vi "CRYASIO Play Buffer.vi"(6 "Gen Idx":u32, 7 "is Main":bool, 8 "Limit":u32, 9 "Buffer Amount":u32, 10 "Buffer Index":u32, 11 "Data Array":sgl[](array[numeric])) -> (0 "Buffer Amount Out":u32, 1 "Buffer Index Out":u32)   [LabVIEW 2013]
uses:
  CRYMisc vis settings global.vi
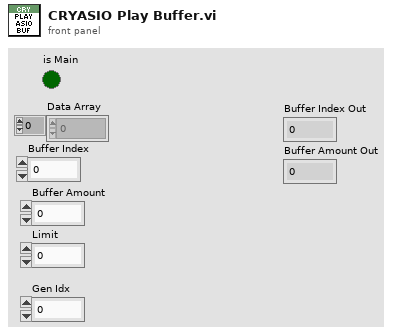
[diagram p1: front panel]
types:
  T1 = cluster{"Gen Idx":i32, "Chn Idx":i32, "Data":sgl[]}[]
  T2 = cluster{"Gen Idx":i32, "Chn Idx":i32, "Data":sgl[]}
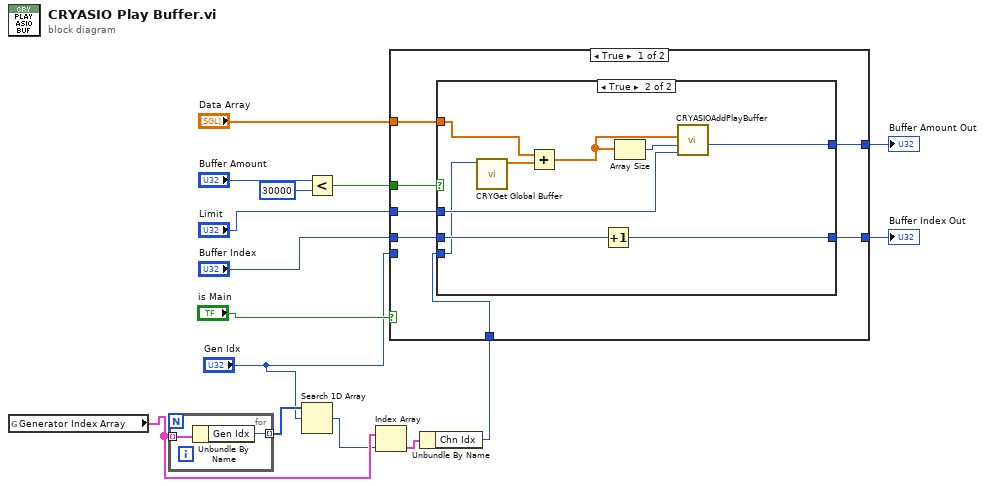
[diagram p0: block diagram]
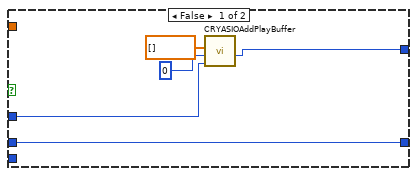
[diagram p2: hidden frame]
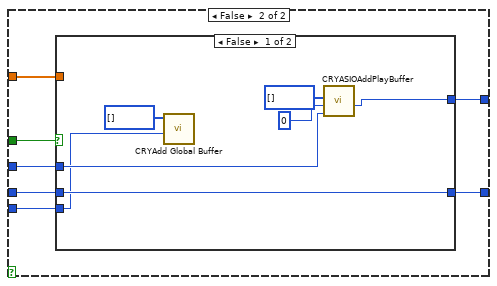
[diagram p3: hidden frame]
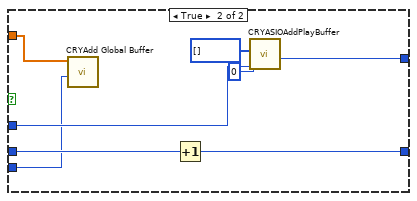
[diagram p4: hidden frame]
diagram:
  n1 = global read "CRYMisc vis settings global.vi" "Generator Index Array"() -> (w4:T1)
  n2 = for {
    tunnel: w4 -> [w17] mode=indexing
    tunnel: [w16] -> w6 mode=indexing
    n3 = Unbundle By Name(w17) -> ("Gen Idx"=w16:i32)
  }
  n4 = Search 1D Array(1D array=w6, element="Gen Idx") -> (index of element=w3:i32)  [unwired: 1 in]
  n5 = Less?(x="Buffer Amount", y=u32 30000) -> (x < y?=w13:bool)
  n6 = Index Array(array=w4, index=w3) -> (element=w2:T2)
  n7 = Unbundle By Name(w2) -> ("Chn Idx"=w1:i32)
  n8 = case shown="True" "is Main" {
    tunnel: w13 -> [w24 w45]
    tunnel: "Data Array" -> [w23 w44]
    tunnel: "Buffer Index" -> [w22 w43]
    tunnel: [w21 w42] -> w10
    tunnel: "Limit" -> [w20 w41]
    tunnel: [w19 w40] -> w8
    tunnel: "Gen Idx" -> [_ w39]
    tunnel: w1 -> [w18 _]
    frame True {
      n9 = case shown="True" w24 {
        tunnel: w23 -> [_ w31]
        tunnel: w22 -> [w29 w38]
        tunnel: [w29 w37] -> w21
        tunnel: w20 -> [w26 w35]
        tunnel: [w25 w34] -> w19
        tunnel: w18 -> [_ w33]
        frame False {
          n10 = call "CRYASIOAddPlayBuffer.vi"("Limit"=w26, "Data Length"=0, "pData"=sgl[] []) -> ("Buffer Amount"=w25:i32)  [unwired: 5 in, 2 out]
        }
        frame True {
          n11 = call "CRYGet Global Buffer.vi"("Chn Idx"=w33) -> ("Global Buffer Out"=w32:sgl[])  [unwired: 8 in, 1 out]
          n12 = Add(x=w31, y=w32) -> (x+y=w30:sgl[])
          n13 = Increment(x=w38) -> (x+1=w37:u32)
          n14 = Array Size(array=w30) -> (size(s)=w36:i32)
          n15 = call "CRYASIOAddPlayBuffer.vi"("Limit"=w35, "Data Length"=w36, "pData"=w30) -> ("Buffer Amount"=w34:i32)  [unwired: 5 in, 2 out]
        }
      }
    }
    frame False {
      n16 = case shown="False" w45 {
        tunnel: w44 -> [_ w56]
        tunnel: w43 -> [w52 w60]
        tunnel: [w52 w59] -> w42
        tunnel: w41 -> [w49 w58]
        tunnel: [w48 w57] -> w40
        tunnel: w39 -> [w47 w55]
        frame False {
          n17 = call "CRYAdd Global Buffer.vi"("Gen Idx"=w47, "Data"=i32[] []) -> ()  [unwired: 10 in]
          n18 = call "CRYASIOAddPlayBuffer.vi"("Limit"=w49, "Data Length"=0, "pData"=i32[] []) -> ("Buffer Amount"=w48:i32)  [unwired: 5 in, 2 out]
        }
        frame True {
          n19 = call "CRYAdd Global Buffer.vi"("Gen Idx"=w55, "Data"=w56) -> ()  [unwired: 10 in]
          n20 = Increment(x=w60) -> (x+1=w59:u32)
          n21 = call "CRYASIOAddPlayBuffer.vi"("Limit"=w58, "Data Length"=0, "pData"=i32[] []) -> ("Buffer Amount"=w57:i32)  [unwired: 5 in, 2 out]
        }
      }
    }
  }
  "Buffer Index Out" <- w10
  "Buffer Amount Out" <- w8
